vi "Memory.vi"(11 "memory":u8[](array[numeric])) -> (3 "output cluster":T1)   [LabVIEW 2015, in "PolyVIEW.lvclass"]
uses:
  PolyVIEW.lvclass
  Memory.ctl
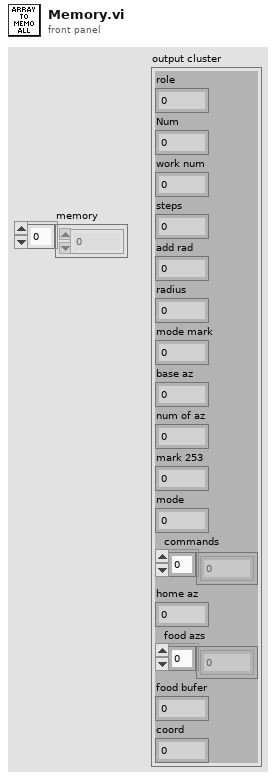
[diagram p1: front panel]
types:
  T1 = typedef "PolyVIEW.lvclass/Memory.ctl" = cluster{"role":i32, "Num":i32, "work num":i32, "steps":dbl, "add rad":i32, "radius":dbl, "mode mark":u32, "base az":dbl, "num of az":u32, "mark 253":u32, "mode":u32, "commands":i32[], "home az":dbl, "food azs":dbl[], "food bufer":dbl, "coord":cdb}
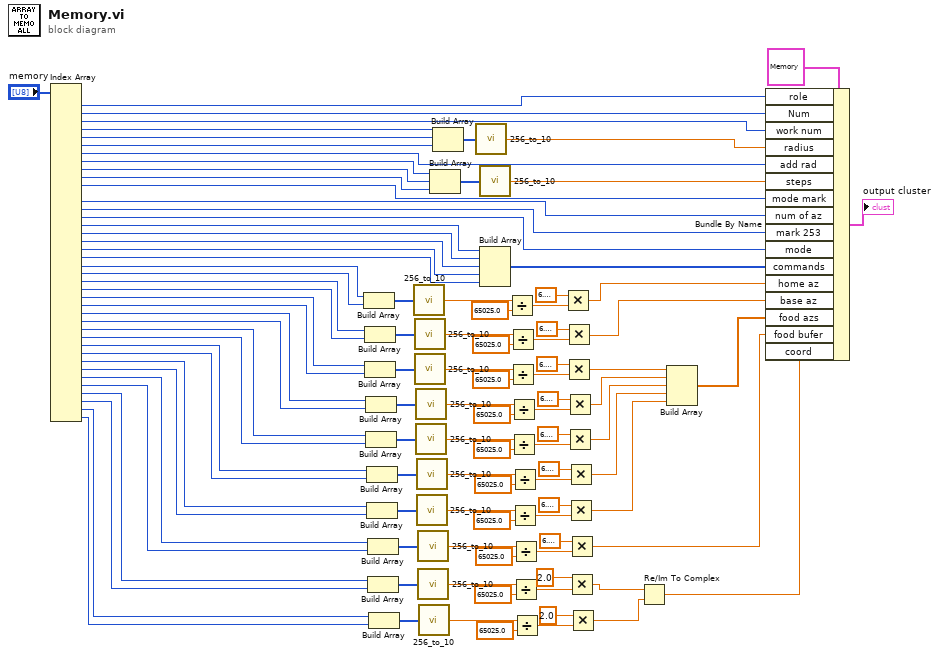
[diagram p0: block diagram]
diagram:
  n1 = Index Array(array="memory") -> (element #1=w95:u8, element #2=w96:u8, element #3=w99:u8, element #4=w100:u8, element #5=w98:u8, element #6=w97:u8, element #7=w103:u8, element #8=w104:u8, element #9=w105:u8, element #10=w106:u8, element #11=w108:u8, element #13=w83:u8, element #14=w92:u8, element #15=w91:u8, element #16=w90:u8, element #17=w89:u8, element #18=w88:u8, element #19=w87:u8, element #20=w86:u8, element #21=w81:u8, element #22=w80:u8, element #23=w69:u8, element #24=w68:u8, element #25=w61:u8, element #26=w60:u8, element #27=w39:u8, element #28=w38:u8, element #29=w37:u8, element #30=w36:u8, element #31=w35:u8, element #32=w34:u8, element #33=w33:u8, element #34=w32:u8, element #35=w20:u8, element #36=w19:u8, element #37=w9:u8, element #38=w8:u8, element #39=w7:u8, element #40=w6:u8)  [unwired: 40 in, 1 out]
  n2 = Build Array(w81, w80) -> (w82:u8[])
  n3 = Build Array(w69, w68) -> (w70:u8[])
  n4 = Build Array(w61, w60) -> (w62:u8[])
  n5 = Build Array(w39, w38) -> (w55:u8[])
  n6 = Build Array(w37, w36) -> (w50:u8[])
  n7 = Build Array(w35, w34) -> (w45:u8[])
  n8 = Build Array(w33, w32) -> (w40:u8[])
  n9 = Build Array(w20, w19) -> (w21:u8[])
  n10 = Build Array(w9, w8) -> (w14:u8[])
  n11 = Build Array(w7, w6) -> (w10:u8[])
  n12 = call "256_to_10.vi"("Array"=w82) -> ("Numeric"=w79:dbl)
  n13 = call "256_to_10.vi"("Array"=w70) -> ("Numeric"=w74:dbl)
  n14 = call "256_to_10.vi"("Array"=w62) -> ("Numeric"=w66:dbl)
  n15 = call "256_to_10.vi"("Array"=w55) -> ("Numeric"=w59:dbl)
  n16 = call "256_to_10.vi"("Array"=w50) -> ("Numeric"=w54:dbl)
  n17 = call "256_to_10.vi"("Array"=w45) -> ("Numeric"=w49:dbl)
  n18 = call "256_to_10.vi"("Array"=w40) -> ("Numeric"=w44:dbl)
  n19 = call "256_to_10.vi"("Array"=w21) -> ("Numeric"=w25:dbl)
  n20 = call "256_to_10.vi"("Array"=w14) -> ("Numeric"=w17:dbl)
  n21 = call "256_to_10.vi"("Array"=w10) -> ("Numeric"=w13:dbl)
  n22 = Build Array(w104, w105, w106) -> (w107:u8[])
  n23 = Build Array(w100, w98, w97) -> (w101:u8[])
  n24 = call "256_to_10.vi"("Array"=w101) -> ("Numeric"=w102:dbl)
  n25 = call "256_to_10.vi"("Array"=w107) -> ("Numeric"=w84:dbl)
  n26 = Build Array(w90, w89, w88, w87, w86) -> (w85:u8[])
  n27 = Divide(x=w79, y=65025.0) -> (x/y=w76:dbl)
  n28 = Divide(x=w74, y=65025.0) -> (x/y=w71:dbl)
  n29 = Divide(x=w66, y=65025.0) -> (x/y=w63:dbl)
  n30 = Divide(x=w59, y=65025.0) -> (x/y=w56:dbl)
  n31 = Divide(x=w54, y=65025.0) -> (x/y=w51:dbl)
  n32 = Divide(x=w49, y=65025.0) -> (x/y=w46:dbl)
  n33 = Divide(x=w44, y=65025.0) -> (x/y=w41:dbl)
  n34 = Divide(x=w25, y=65025.0) -> (x/y=w22:dbl)
  n35 = Divide(x=w17, y=65025.0) -> (x/y=w15:dbl)
  n36 = Divide(x=w13, y=65025.0) -> (x/y=w11:dbl)
  n37 = Multiply(x=6.283185307179586, y=w76) -> (x*y=w75:dbl)
  n38 = Multiply(x=6.283185307179586, y=w71) -> (x*y=w67:dbl)
  n39 = Multiply(x=6.283185307179586, y=w63) -> (x*y=w27:dbl)
  n40 = Multiply(x=6.283185307179586, y=w56) -> (x*y=w28:dbl)
  n41 = Multiply(x=6.283185307179586, y=w51) -> (x*y=w29:dbl)
  n42 = Multiply(x=6.283185307179586, y=w46) -> (x*y=w30:dbl)
  n43 = Multiply(x=6.283185307179586, y=w41) -> (x*y=w31:dbl)
  n44 = Multiply(x=6.283185307179586, y=w22) -> (x*y=w18:dbl)
  n45 = Multiply(x=2.0, y=w15) -> (x*y=w3:dbl)
  n46 = Multiply(x=2.0, y=w11) -> (x*y=w2:dbl)
  n47 = Re/Im To Complex(1:w2, 2:w3) -> (0:w1:cdb)
  n48 = Build Array(w27, w28, w29, w30, w31) -> (w26:dbl[])
  n49 = Bundle By Name(cluster=T1 {"role"=0, "Num"=0, "work num"=0, "steps"=0.0, "add rad"=0, "radius"=0.0, "mode mark"=0, "base az"=0.0, "num of az"=0, "mark 253"=0, "mode"=0, "commands"=[], "home az"=0.0, "food azs"=[], "food bufer"=0.0, "coord"=0.0+0.0i}, "role"=w95, "Num"=w96, "work num"=w99, "radius"=w102, "add rad"=w103, "steps"=w84, "mode mark"=w108, "num of az"=w83, "mark 253"=w92, "mode"=w91, "commands"=w85, "home az"=w75, "base az"=w67, "food azs"=w26, "food bufer"=w18, "coord"=w1) -> (→"output cluster":T1)
